vi "220402_STEPN_maltiReader.vi"() -> ()   [LabVIEW 2016]
uses:
  <vilib>/Utility/file.llb/Write Delimited Spreadsheet (string).vi
panel:
  in  "Mode":enum16{"walking", "Repair", "wallet Balance"}(ring)
  out "String N":string[](array[string])
  out "i _moji count":i32[](array[numeric])
  out "Total Moji Count":i32[](array[numeric])
  out "finish time(s)":dbl format="%.1f"
  out "average time(s)":dbl format="%#.1g"
  out "total time(s)":dbl format="%.1f"
  out "elapsed time(s)":dbl[](array[numeric]) format="%.2g"
  out "sumtime(s)":dbl format="%.1g"
  out "ratio(%)":dbl[](array[numeric]) format="%.1g"
  out "数値":i32
  out "dataN":i32
  out "reading path":path=path "G:/マイドライブ/STEPN_walking/IMG_5909.PNG" caption="PNG single path"
  out "Save filename":path
  in  "new file path (Not A Path if cancelled)":path=path "G:/マイドライブ/STEPN/STEPN_csv" caption="Save to Path"
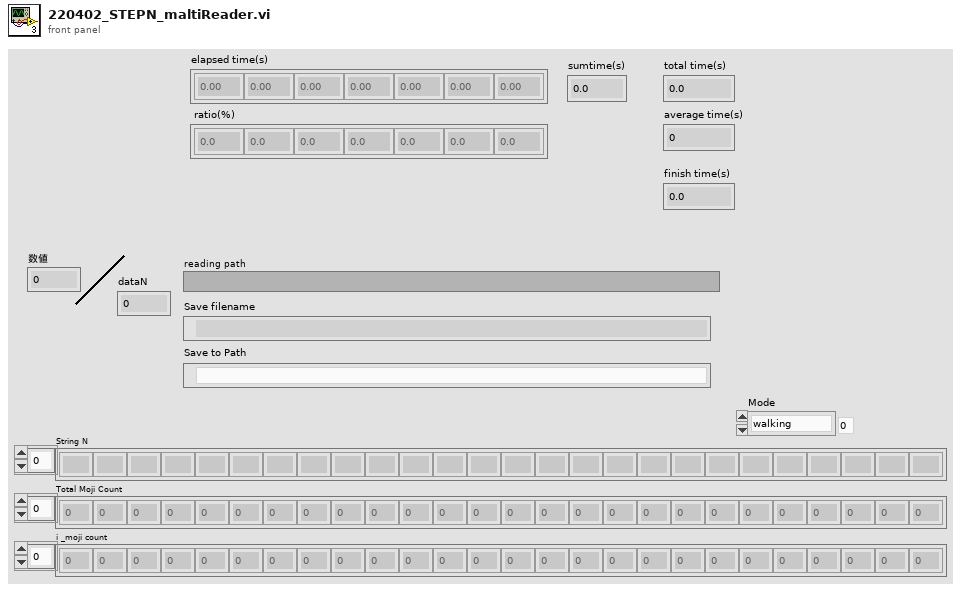
[diagram p1: front panel]
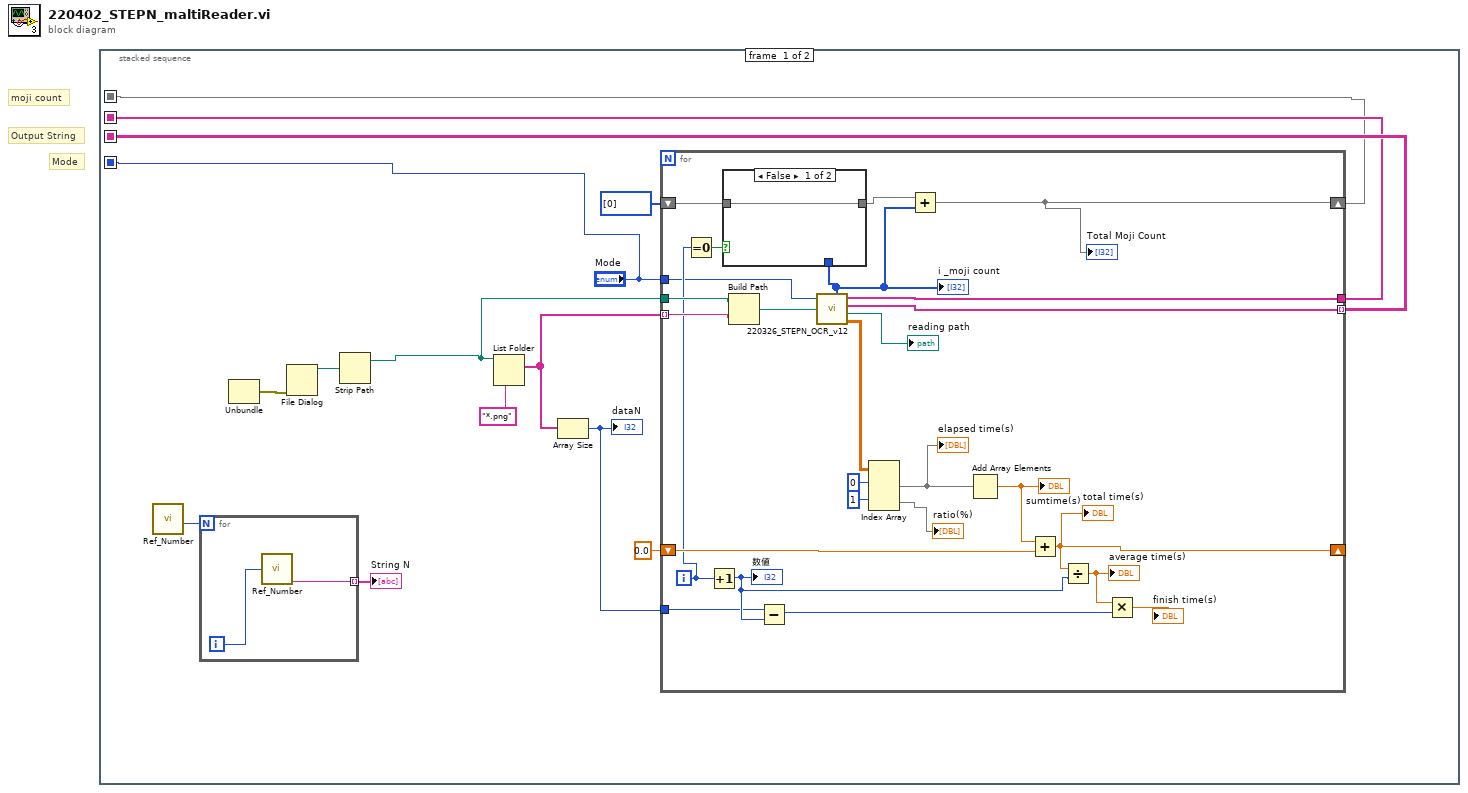
[diagram p0: block diagram]
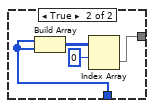
[diagram p2: hidden frame]
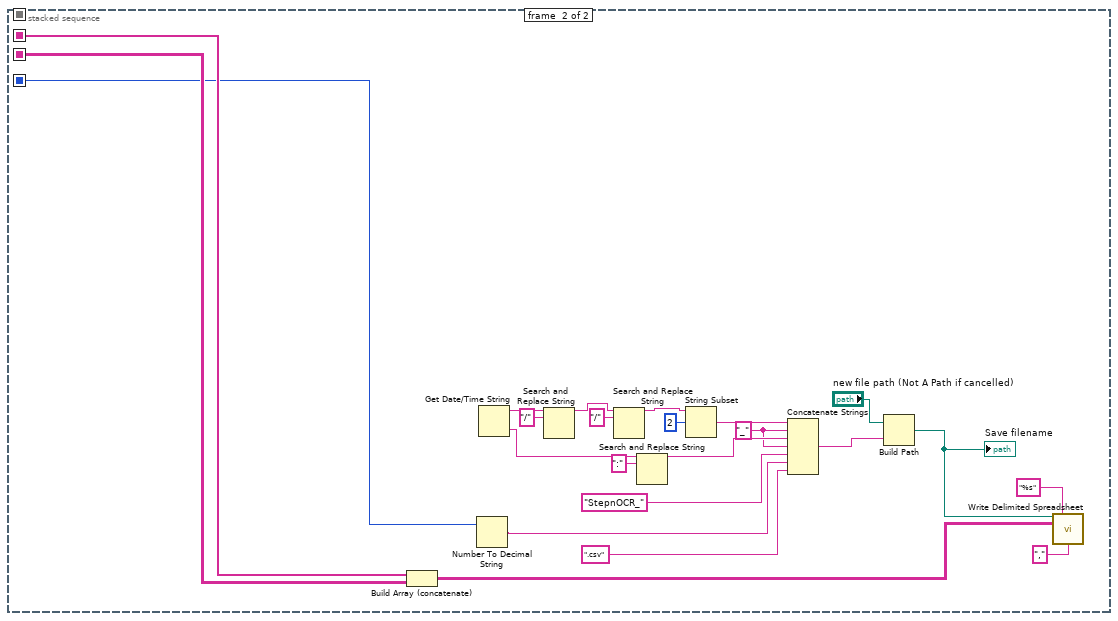
[diagram p3: hidden frame]
diagram:
  # "Mode"
  # "moji count"
  # "Output String"
  n1 = stacked-sequence {
    seq-local: [w10 _] -> [_ w52]
    seq-local: [w9 _] -> [_ w53]
    seq-local: [w4 _] -> [_ _]
    seq-local: ["Mode" _] -> [_ w50]
    frame #0 {
      n2 = call "Ref_Number.vi"() -> ("total ref."=w3:i32)  [unwired: 1 in, 3 out]
      n3 = for {
        N: w3 -> [_]
        tunnel: [w15] -> w2 mode=indexing
        i -> [w16]
        n4 = call "Ref_Number.vi"("inform N."=w16) -> ("Output string"=w15:string)  [unwired: 3 out]
      }
      "String N" <- w2
      n5 = File Dialog() -> (0:w13:errorcluster, 3:w12:path)  [unwired: 7 in, 2 out]
      n6 = Unbundle(w13) -> ()  [unwired: 3 out]
      n7 = Strip Path(path=w12) -> (stripped path=w11:path)  [unwired: 1 out]
      n8 = List Folder(path=w11, pattern="*.png") -> (filenames=w8:string[])  [unwired: 2 in, 3 out]
      n9 = Array Size(array=w8) -> (size(s)=w6:i32)
      "dataN" <- w6
      n10 = for {
        tunnel: w11 -> [w42]
        tunnel: w8 -> [w41] mode=indexing
        tunnel: [w39] -> w10 mode=indexing
        tunnel: [w37] -> w9
        shift-right: [w29] -> _
        shift-left: 0.0 -> [w30]
        tunnel: w6 -> [w27]
        shift-right: [w23] -> w4
        shift-left: i32[] [0] -> [w20]
        tunnel: "Mode" -> [w17]
        i -> [w21]
        n11 = Equal To 0?(x=w21) -> (x = 0?=w22:bool)
        n12 = Increment(x=w21) -> (x+1=w28:i32)
        "数値" <- w28
        n13 = Build Path(base path=w42, name or relative path=w41) -> (appended path=w40:path)
        n14 = Subtract(x=w27, y=w28) -> (x-y=w25:i32)
        n15 = call "220326_STEPN_OCR_v12.vi"("Mode"=w17, "path to PNG file"=w40) -> ("item"=w37:string[], "Output String"=w39:string[], "reading path"=→"reading path":path, "elapsed time(s)"=w36:dbl[][], "moji N"=w18:i32[])  [unwired: 1 in]
        "i _moji count" <- w18
        n16 = case shown="False" w22 {
          tunnel: w20 -> [w43 _]
          tunnel: [w43 w45] -> w19
          tunnel: w18 -> [_ w47]
          frame False {
          }
          frame True {
            n17 = Build Array(w47, w47) -> (w46:i32[][])
            n18 = Index Array(array=w46, index (row)=0 ("指標 （行）")) -> (element=w45:i32[])  [unwired: 1 in]
          }
        }
        n19 = Index Array(array=w36, index (row) #1=0 ("指標 （行）"), index (row) #2=1 ("指標 （行）")) -> (element #1=w34:dbl[], element #2=→"ratio(%)":dbl[])  [unwired: 2 in]
        "elapsed time(s)" <- w34
        n20 = Add(x=w19, y=w18) -> (x+y=w23:i32[])
        "Total Moji Count" <- w23
        n21 = Add Array Elements(numeric array=w34) -> (sum=w31:dbl)
        "sumtime(s)" <- w31
        n22 = Add(x=w31, y=w30) -> (x+y=w29:dbl)
        "total time(s)" <- w29
        n23 = Divide(x=w29, y=w28) -> (x/y=w26:dbl)
        "average time(s)" <- w26
        n24 = Multiply(x=w26, y=w25) -> (x*y=→"finish time(s)":dbl)
      }
    }
    frame #1 {
      w59 = "_" ("文字列")
      n25 = Build Array (concatenate)(w53, w52) -> (w51:string[][])
      n26 = Number To Decimal String(number=w50) -> (decimal integer string=w49:string)  [unwired: 1 in]
      n27 = Get Date/Time String() -> (date string=w70:string, time string=w66:string)  [unwired: 3 in]
      n28 = Search and Replace String(input string=w70, search string="/" ("検索文字列")) -> (result string=w63:string)  [unwired: 6 in, 3 out]
      n29 = Search and Replace String(input string=w63, search string="/" ("検索文字列")) -> (result string=w62:string)  [unwired: 6 in, 3 out]
      n30 = Search and Replace String(input string=w66, search string=":" ("検索文字列")) -> (result string=w60:string)  [unwired: 6 in, 3 out]
      n31 = String Subset(string=w62, offset (0)=2 ("オフセット（0）")) -> (substring=w65:string)  [unwired: 1 in]
      n32 = Concatenate Strings(w65, w59, w60, w59, "StepnOCR_", w49, ".csv") -> (w56:string)
      n33 = Build Path(base path="new file path (Not A Path if cancelled)", name or relative path=w56) -> (appended path=w54:path)
      "Save filename" <- w54
      n34 = call-poly <vilib>:"Write Delimited Spreadsheet.vi"("file path (dialog if empty)"=w54, "format (%s)"="%s", "2D data"=w51, "delimiter (\\t)"="," ("delimiter (\\t)")) -> ()  [unwired: 10 in, 2 out]
    }
  }
